vi "FlyWheelLookup.vi"(11 "Inputs_All":T1) -> ()   [LabVIEW 2011]
uses:
  Inputs_All.ctl
  Flywheel/Inputs_FlyWheel.ctl
  tankdrive/Input_Wheel_Speeds.ctl
  Conveyor/Conveyor_input.ctl
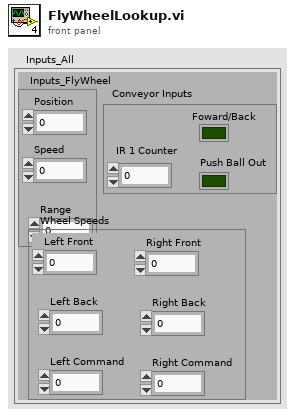
[diagram p1: front panel]
types:
  T1 = typedef "Inputs_All.ctl" = cluster{"Inputs_FlyWheel":T2, "Wheel Speeds":T3, "Conveyor Inputs":T4}
  T2 = typedef "Inputs_FlyWheel.ctl" = cluster{"Position":dbl, "Speed":dbl, "Range":dbl}
  T3 = typedef "Input_Wheel_Speeds.ctl" = cluster{"Left Front":dbl, "Right Front":dbl, "Left Back":dbl, "Right Back":dbl, "Left Command":dbl, "Right Command":dbl}
  T4 = typedef "Conveyor_input.ctl" = cluster{"Foward/Back":bool, "IR 1 Counter":i32, "Push Ball Out":bool}
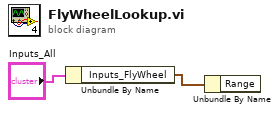
[diagram p0: block diagram]
diagram:
  n1 = Unbundle By Name("Inputs_All") -> ("Inputs_FlyWheel"=w1:T2)
  n2 = Unbundle By Name(w1) -> ()  [unwired: 1 out]
